vi "MEMR-Copy Database.vi"() -> ()   [LabVIEW 2015]
panel:
  in  "Database":path=path "C:/Data/MEMR Analysis/database MEMR.csv"
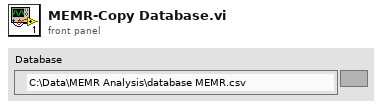
[diagram p1: front panel]
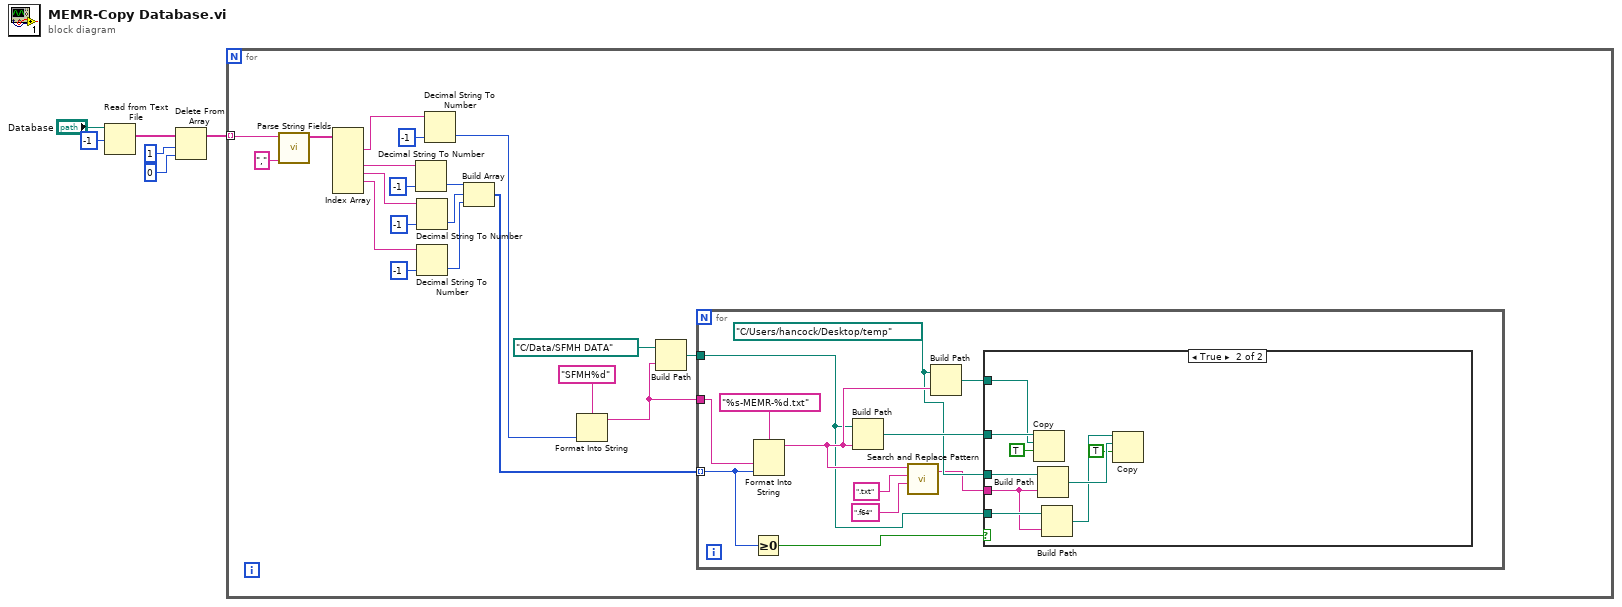
[diagram p0: block diagram]
diagram:
  n1 = Read from Text File(file (use dialog)="Database", count=-1) -> (text=w4:string[])  [unwired: 2 in, 3 out]
  n2 = Delete From Array(array=w4, length=1, index=0) -> (array with subset deleted=w1:string[])  [unwired: 1 out]
  n3 = for {
    tunnel: w1 -> [w26] mode=indexing
    n4 = call "Parse String Fields.vi"("Separator"=",", "String"=w26) -> ("Fields"=w24:string[])  [unwired: 8 in, 1 out]
    n5 = Index Array(array=w24) -> (element #1=w8:string, element #3=w23:string, element #4=w19:string, element #5=w18:string)  [unwired: 6 in, 2 out]
    n6 = Decimal String To Number(string=w23, default (0L)=-1 ("default (0 I32)")) -> (number=w17:i32)  [unwired: 1 in, 1 out]
    n7 = Decimal String To Number(string=w19, default (0L)=-1 ("default (0 I32)")) -> (number=w16:i32)  [unwired: 1 in, 1 out]
    n8 = Decimal String To Number(string=w18, default (0L)=-1 ("default (0 I32)")) -> (number=w15:i32)  [unwired: 1 in, 1 out]
    n9 = Decimal String To Number(string=w8, default (0L)=-1 ("default (0 I32)")) -> (number=w7:i32)  [unwired: 1 in, 1 out]
    n10 = Build Array(w17, w16, w15) -> (w10:i32[])
    n11 = Format Into String(format string="SFMH%d", w7) -> (resulting string=w11:string)  [unwired: 2 in, 1 out]
    n12 = Build Path(base path=path "C:/Data/SFMH DATA", name or relative path=w11) -> (appended path=w12:path)
    n13 = for {
      tunnel: w12 -> [w27]
      tunnel: w10 -> [w36] mode=indexing
      tunnel: w11 -> [w37]
      w29 = path "C:/Users/hancock/Desktop/temp"
      n14 = Greater Or Equal To 0?(x=w36) -> (x >= 0?=w33:bool)
      n15 = Format Into String(format string="%s-MEMR-%d.txt", w37, w36) -> (resulting string=w30:string)  [unwired: 2 in, 1 out]
      n16 = Build Path(base path=w27, name or relative path=w30) -> (appended path=w35:path)
      n17 = call <vilib>:"Search and Replace Pattern.vi"("string"=w30, "regular expression (\"\")"=".txt" ("regular expression (\"\")"), "replace string (\"\")"=".f64" ("replace string (\"\")")) -> ("result string"=w28:string)  [unwired: 2 in, 1 out]
      n18 = Build Path(base path=w29, name or relative path=w30) -> (appended path=w34:path)
      n19 = case shown="True" w33 {
        tunnel: w35 -> [_ w47]
        tunnel: w34 -> [_ w46]
        tunnel: w29 -> [_ w44]
        tunnel: w28 -> [_ w42]
        tunnel: w27 -> [_ w43]
        frame False {
        }
        frame True {
          n20 = Copy(9:TRUE ("overwrite (F)"), 10:w46, 11:w47) -> ()  [unwired: 2 in, 3 out]
          n21 = Build Path(base path=w44, name or relative path=w42) -> (appended path=w41:path)
          n22 = Build Path(base path=w43, name or relative path=w42) -> (appended path=w40:path)
          n23 = Copy(9:TRUE ("overwrite (F)"), 10:w41, 11:w40) -> ()  [unwired: 2 in, 3 out]
        }
      }
    }
  }
